vi "failure3.vi"() -> ()   [LabVIEW 2018]
panel:
  in  "run time":dbl
  in  "Name":string
  in  "Scores":dbl
  out "Table":string[][](table)
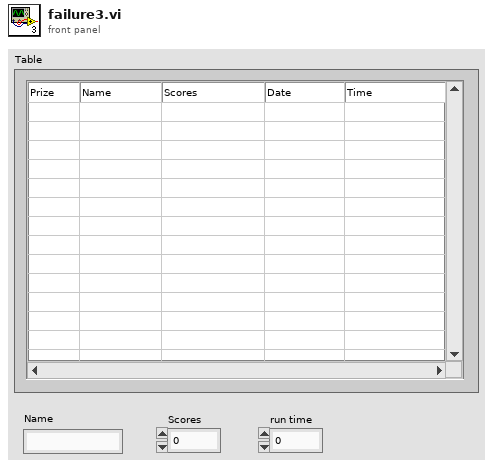
[diagram p1: front panel]
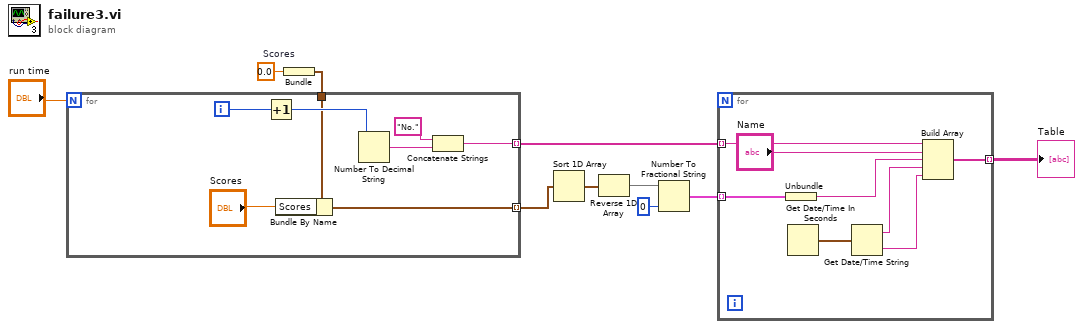
[diagram p0: block diagram]
diagram:
  w4 = 0.0  # Scores
  n1 = Bundle("Scores"=w4) -> (w3:cluster{"Scores":dbl})  [unwired: 1 in]
  n2 = for {
    N: "run time" -> [_]
    tunnel: [w14] -> w9 mode=indexing
    tunnel: w3 -> [w13]
    tunnel: [w11] -> w2 mode=indexing
    i -> [w18]
    n3 = Increment(x=w18) -> (x+1=w17:i32)
    n4 = Bundle By Name(cluster=w13, "Scores"="Scores") -> (w11:cluster{"Scores":dbl})
    n5 = Number To Decimal String(number=w17) -> (decimal integer string=w16:string)  [unwired: 1 in]
    n6 = Concatenate Strings("No." ("string"), w16) -> (w14:string)
  }
  n7 = Sort 1D Array(array=w2) -> (sorted array=w10:cluster{"Scores":dbl}[])
  n8 = Reverse 1D Array(array=w10) -> (reversed array=w8:cluster{"Scores":dbl}[])
  n9 = Number To Fractional String(number=w8, precision (6)=i16 0) -> (F-format string=w6:cluster{"Scores":string}[])  [unwired: 2 in]
  n10 = for {
    tunnel: w9 -> [w25] mode=indexing
    tunnel: w6 -> [w26] mode=indexing
    tunnel: [w19] -> w1 mode=indexing
    n11 = Unbundle(w26) -> ("Scores"=w20:string)
    n12 = Get Date/Time In Seconds() -> (seconds since 1Jan1904=w23:timestamp)
    n13 = Get Date/Time String(seconds (now)=w23) -> (date string=w22:string, time string=w21:string)  [unwired: 2 in]
    n14 = Build Array(w25, "Name", w20, w22, w21) -> (w19:string[])
  }
  "Table" <- w1
